vi "Write Pulse File.vi"(8 "error in (no error)":errorcluster, 9 "Open plot after pulse":bool, 10 "Pulse File":path, 11 "Monitor-Pulse in":refnum<class "LabActor.lvclass">) -> (0 "error out":errorcluster, 3 "Monitor-Pulse out":refnum<class "LabActor.lvclass">)   [LabVIEW 2018, in "LabActor.lvclass"]
uses:
  LabActor.lvclass
  Plots/Plot types.ctl
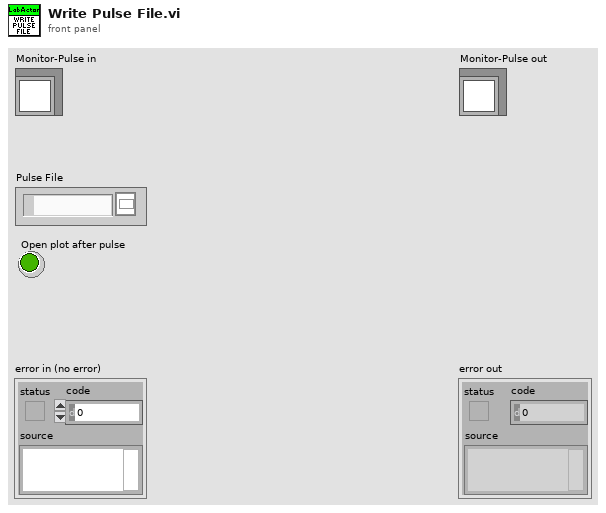
[diagram p1: front panel]
types:
  T1 = typedef "Plot types.ctl" = enum16{"Waveform Plot", "XY Plot", "Full XY"}
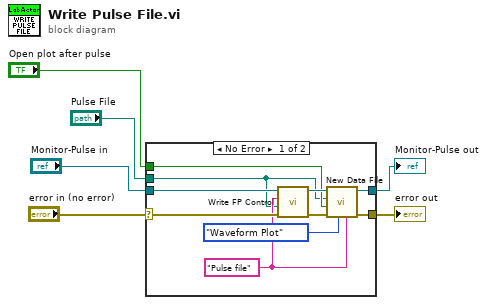
[diagram p0: block diagram]
diagram:
  n1 = case shown="No Error" "error in (no error)" {
    selector: "error in (no error)" -> [w15 w18]
    tunnel: [w11 w18] -> w5
    tunnel: [w13 w17] -> w3
    tunnel: "Monitor-Pulse in" -> [w16 w17]
    tunnel: "Open plot after pulse" -> [w8 _]
    tunnel: "Pulse File" -> [w7 _]
    frame No Error {
      w9 = "Pulse file" ("Control Name")
      n2 = call-dynamic "Write FP Control.vi"("error in (no error)"=w15, "Control Value"=w7, "Control Name"=w9, "Measure Object in"=w16) -> ("error out"=w12:errorcluster, "Measure Object out"=w14:refnum<class "LabActor.lvclass">)  [unwired: 6 in]
      n3 = call-dynamic "New Data File.vi"("Plot group"=w9, "Plot type"=Plot_types."Waveform Plot", "error in (no error)"=w12, "New plot if not open"=w8, "File"=w7, "Application Controller in"=w14) -> ("error out"=w11:errorcluster, "Application Controller out"=w13:refnum<class "LabActor.lvclass">)  [unwired: 4 in]
    }
    frame Error {
    }
  }
  "error out" <- w5
  "Monitor-Pulse out" <- w3
